vi "JoyEventHandler.vi"(11 "UiDefinition":T1) -> ()   [LabVIEW 2020]
uses:
  UIReferences.ctl
  C:/Users/User/Desktop/Automation/NextVersion2/LabviewDXFViewer/bin/Release/LabviewDXFViewer.exe
  LabviewDXFViewer/bin/Release/LabviewDXFViewer.exe
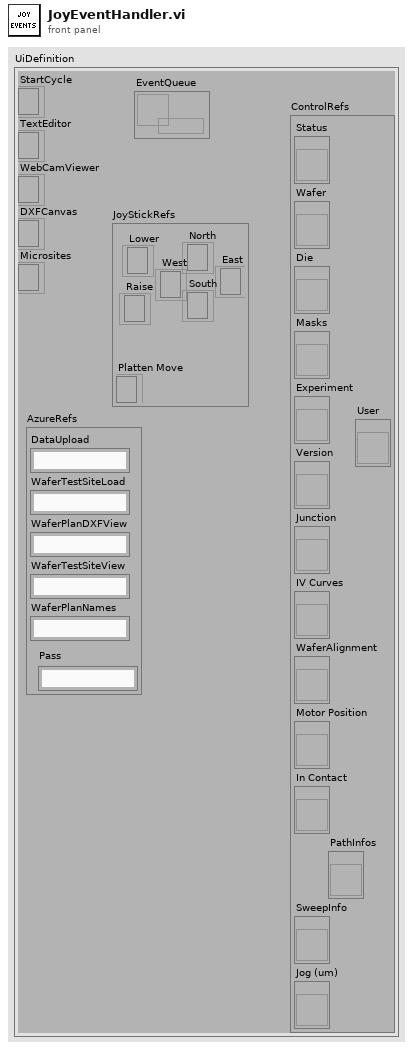
[diagram p1: front panel]
types:
  T1 = typedef "UIReferences.ctl" = cluster{"StartCycle":refnum<k24>, "TextEditor":refnum<k24>, "WebCamViewer":refnum<k24>, "DXFCanvas":refnum<k24>, "Microsites":refnum<k24>, "JoyStickRefs":cluster{"North":refnum<k24>, "Lower":refnum<k24>, "Raise":refnum<k24>, "Platten Move":refnum<k24>, "West":refnum<k24>, "East":refnum<k24>, "South":refnum<k24>}, "AzureRefs":cluster{"DataUpload":string, "WaferTestSiteLoad":string, "WaferPlanDXFView":string, "WaferTestSiteView":string, "WaferPlanNames":string, "Pass":string}, "ControlRefs":cluster{"Status":refnum<vi>, "Wafer":refnum<vi>, "Die":refnum<vi>, "Masks":refnum<vi>, "Experiment":refnum<vi>, "Version":refnum<vi>, "Junction":refnum<vi>, "IV Curves":refnum<vi>, "WaferAlignment":refnum<vi>, "Motor Position":refnum<vi>, "In Contact":refnum<vi>, "SweepInfo":refnum<vi>, "Jog (um)":refnum<vi>, "PathInfos":refnum<vi>, "User":refnum<vi>}, "EventQueue":refnum<queue>}
  T2 = cluster{"North":refnum<k24>, "Lower":refnum<k24>, "Raise":refnum<k24>, "Platten Move":refnum<k24>, "West":refnum<k24>, "East":refnum<k24>, "South":refnum<k24>}
  T3 = cluster{"Wafer Units to microns":dbl, "Rotation Misalign":dbl[], "Scale Misalign":dbl, "Steps Per micron":dbl, "Position 1":i32[], "Chip Orientation":i32, "Position 2":i32[], "Lift Distance":i32, "Position 3":i32[]}
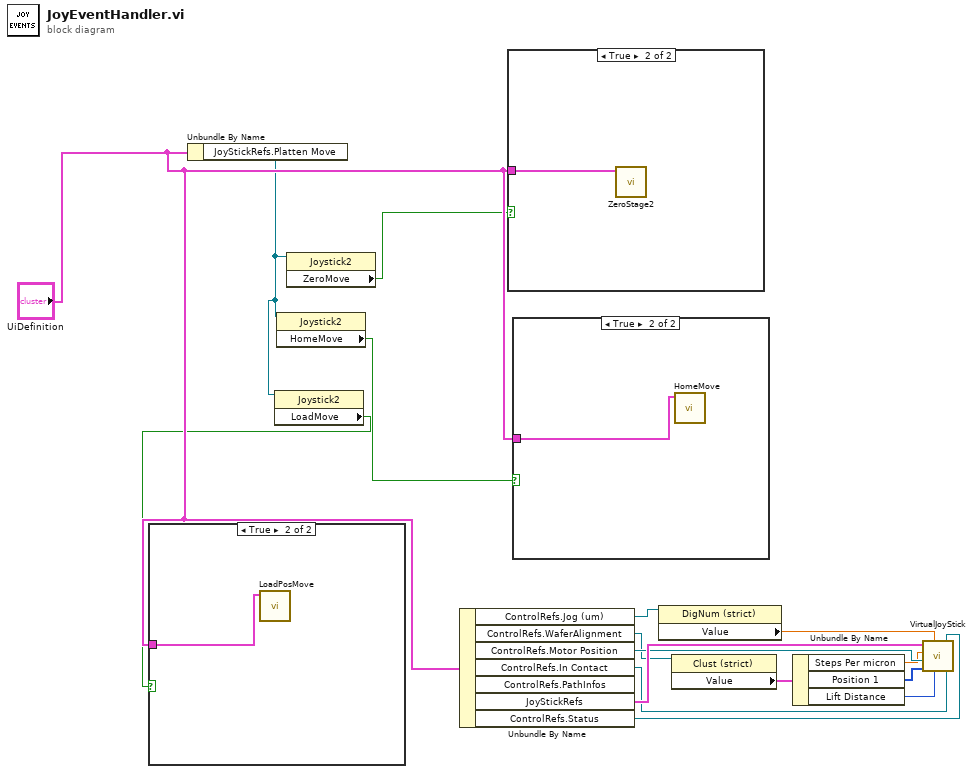
[diagram p0: block diagram]
diagram:
  n1 = Unbundle By Name("UiDefinition") -> ("JoyStickRefs.Platten Move"=w2:refnum<k24>)
  n2 = property class="Joystick2"(reference=w2) -> ("LoadMove"=w4:bool)  [unwired: 1 in, 2 out]
  n3 = case shown="True" w4 {
    tunnel: "UiDefinition" -> [_ w17]
    frame False {
    }
    frame True {
      n4 = call "LoadPosMove.vi"("UiDefinition"=w17) -> ()  [unwired: 11 in]
    }
  }
  n5 = property class="Joystick2"(reference=w2) -> ("HomeMove"=w3:bool)  [unwired: 1 in, 2 out]
  n6 = property class="Joystick2"(reference=w2) -> ("ZeroMove"=w1:bool)  [unwired: 1 in, 2 out]
  n7 = Unbundle By Name("UiDefinition") -> ("ControlRefs.Jog (um)"=w13:refnum<vi>, "ControlRefs.WaferAlignment"=w5:refnum<vi>, "ControlRefs.Motor Position"=w8:refnum<vi>, "ControlRefs.In Contact"=w10:refnum<vi>, "JoyStickRefs"=w12:T2, "ControlRefs.Status"=w15:refnum<vi>)  [unwired: 1 out]
  n8 = case shown="True" w1 {
    tunnel: "UiDefinition" -> [_ w18]
    frame False {
    }
    frame True {
      n9 = call "ZeroStage2.vi"("UiDefinition"=w18) -> ()  [unwired: 11 in]
    }
  }
  n10 = case shown="True" w3 {
    tunnel: "UiDefinition" -> [_ w19]
    frame False {
    }
    frame True {
      n11 = call "HomeMove.vi"("UiDefinition"=w19) -> ()  [unwired: 11 in]
    }
  }
  n12 = property class="DigNum (strict)"(reference=w13) -> ("Value"=w14:dbl)  [unwired: 1 in, 2 out]
  n13 = property class="Clust (strict)"(reference=w5) -> ("Value"=w6:T3)  [unwired: 1 in, 2 out]
  n14 = Unbundle By Name(w6) -> ("Steps Per micron"=w7:dbl, "Position 1"=w9:i32[], "Lift Distance"=w11:i32)
  n15 = call "VirtualJoyStick.vi"("In Contact"=w10, "Status"=w15, "Jog (um) raise"=w11, "Jog (um)"=w14, "Position 1"=w9, "Motor Zero"=w8, "Steps Per micron"=w7, "JoyStickRefs"=w12) -> ()
